vi "纳清叶绿素a电极校准.vi"() -> ()   [LabVIEW 2016, in "斯坦道多参数.lvlib"]
uses:
  <vilib>/Utility/miscctls.llb/LVPointTypeDef.ctl
  <vilib>/Utility/miscctls.llb/LVPositionTypeDef.ctl
  <vilib>/Analysis/NI_AALBase.lvlib
panel:
  out "温度校准参数":sgl
  out "第三点校准值":dbl
  out "标液3":sgl
  out "第二点校准值":dbl
  out "第一点校准值":dbl
  in  "校准停止":bool
  in  "校准启动":bool
  in  "校准模式":enum16{"两点校准", "单点校准", "三点校准"}(ring)=enum."单点校准"
  out "最小值":sgl format="%#.2f"
  out "最大值":sgl format="%#.2f"
  out "波形图表":u16(graph) caption="历史曲线"
  out "mean":dbl caption="均值" format="%#.2f"
  out "standard deviation":dbl caption="标准差" format="%#.2f"
  out "变异系数":dbl format="%#.6f"
  out "测量值":sgl
  out "提示":string
  out "标液2":sgl
  out "标液1":sgl
  out "原始光强数值":u16 caption="信号值"
  out "温度":dbl
  # "叶绿素a电极设定"
  # "℃"
  # "ug/L"
  # "℃"
  # "请选择校准模式:"
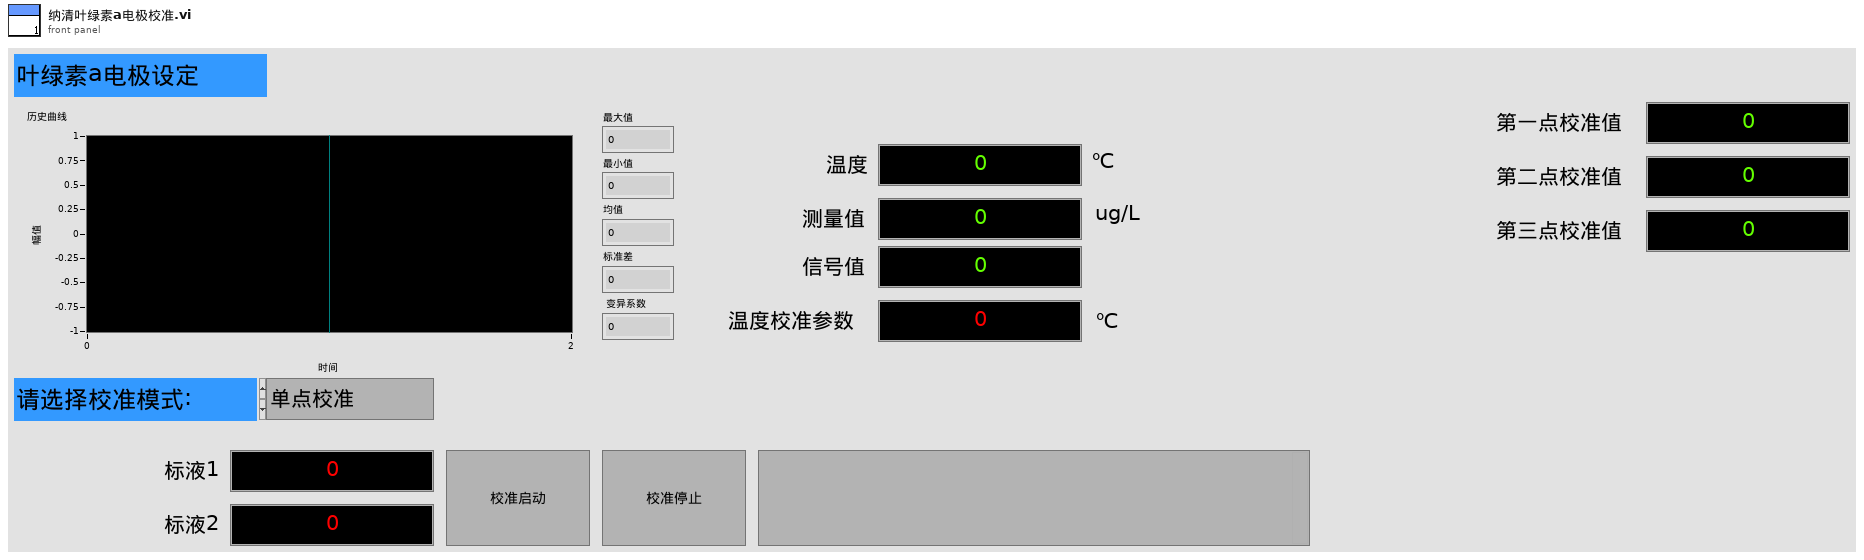
[diagram p1: front panel]
types:
  T1 = typedef "LVPointTypeDef.ctl" = cluster{"Horizontal":i16, "Vertical":i16}
  T2 = typedef "斯坦道多参数.lvlib/校准步骤.ctl" = enum16{"待机", "放置第一点标液", "第一点校准启动", "第一点校准写入", "第一点校准失败", "放置第二点标液", "第二点校准启动", "第二点校准写入", "第二点校准失败", "放置第三点标液", "第三点校准启动", "第三点校准写入", "第三点校准失败", "校准结果写入", "校准结束"}
  T3 = cluster{"报警码":u16, "叶绿素a":sgl, "温度数据":sgl, "原始光强数值":u16, "0X0006_NC":u16, "平均次数":u16, "清扫模式":u16, "清扫次数":u16, "清扫间隔分钟":u16, "0X000B_NC":string, "产品名称":string, "序列号":string, "硬件版本":string, "软件版本":string, "通讯地址":u16, "波特率":u16, "设备类型":u16, "0X0026_NC":string, "0X0030_NC":u16, "第一点原始光强":u16, "第一点校准数据":sgl, "第二点原始光强":u16, "第二点校准数据":sgl, "第三点原始光强":u16, "第三点校准数据":sgl, "探头校准命令":u16, "温度校准参数":sgl, "温度校准命令":u16}
  T4 = typedef "LVPositionTypeDef.ctl" = cluster{"Left":i32, "Top":i32}
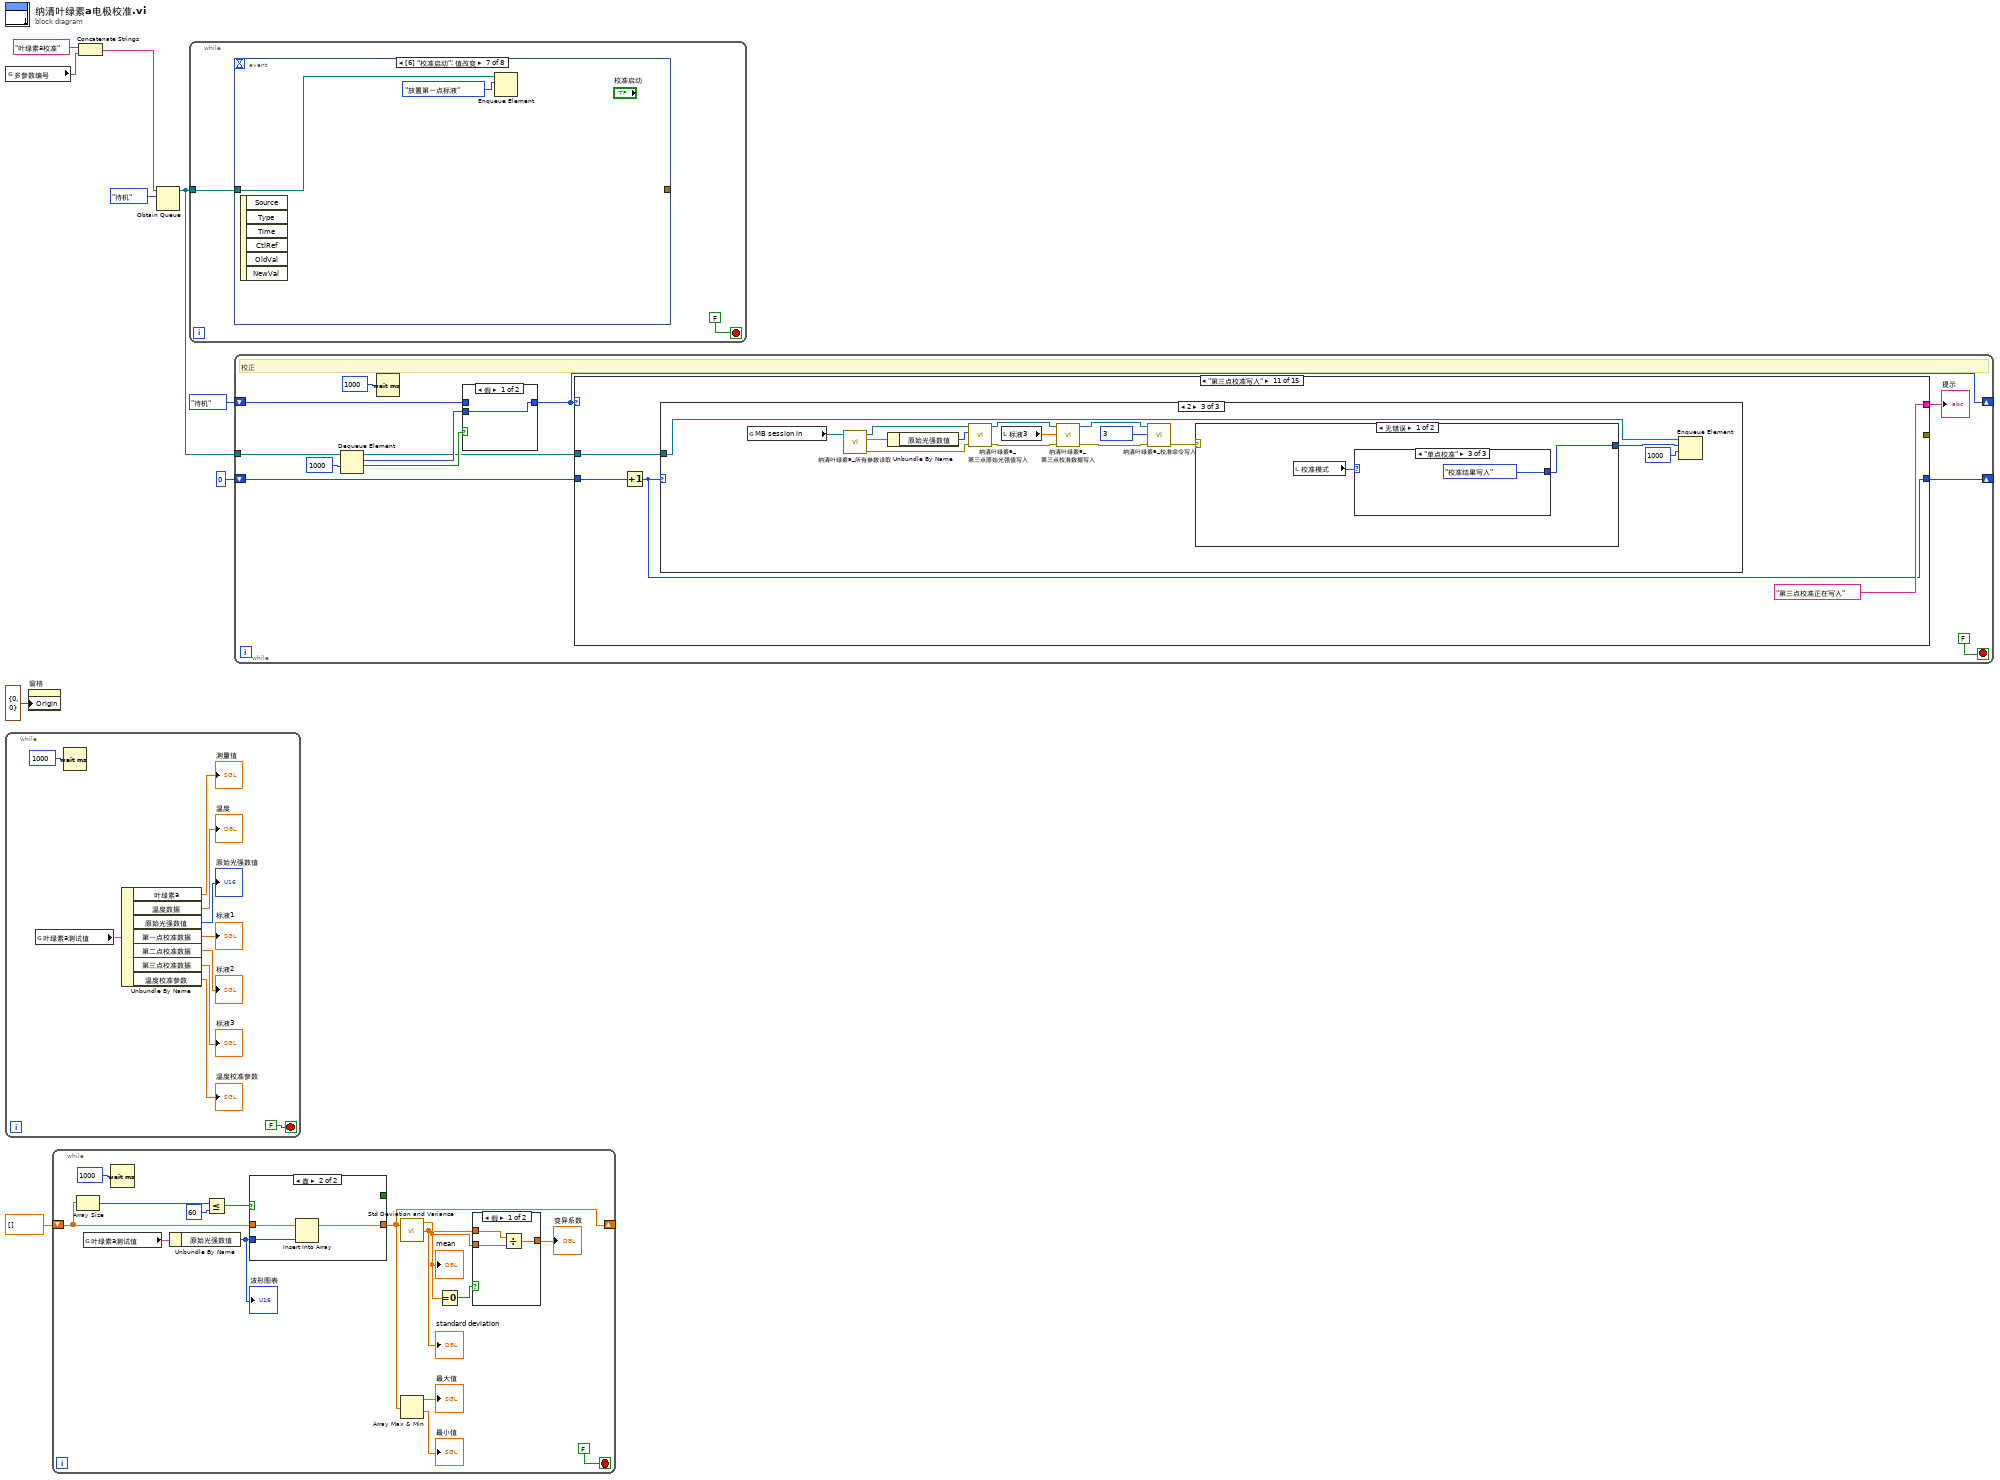
[diagram p0: block diagram]
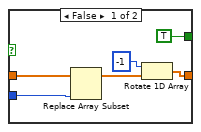
[diagram p3: hidden frame]
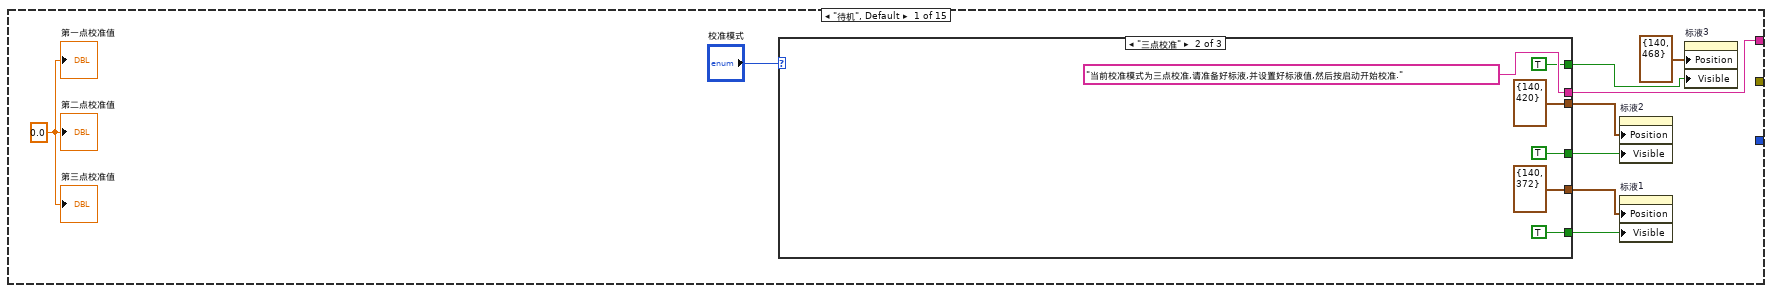
[diagram p5: hidden frame]
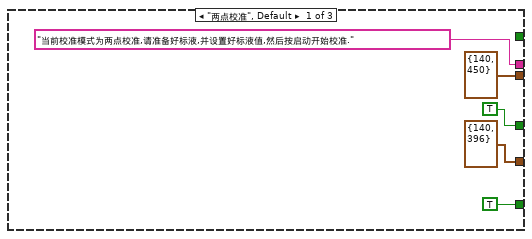
[diagram p6: hidden frame]
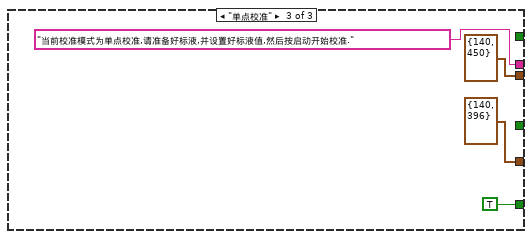
[diagram p7: hidden frame]
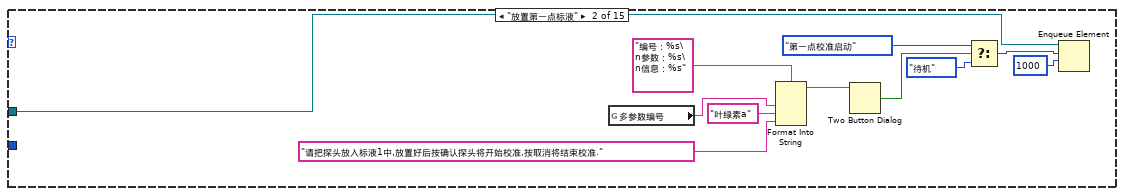
[diagram p8: hidden frame]
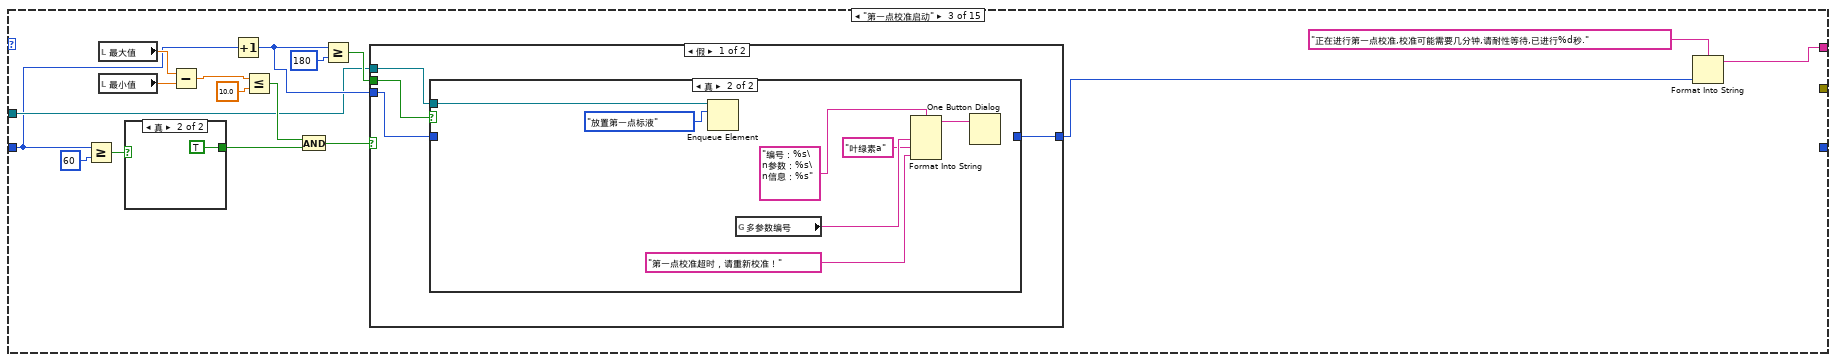
[diagram p9: hidden frame]
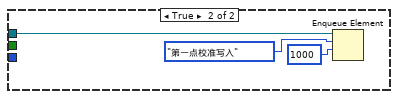
[diagram p11: hidden frame]
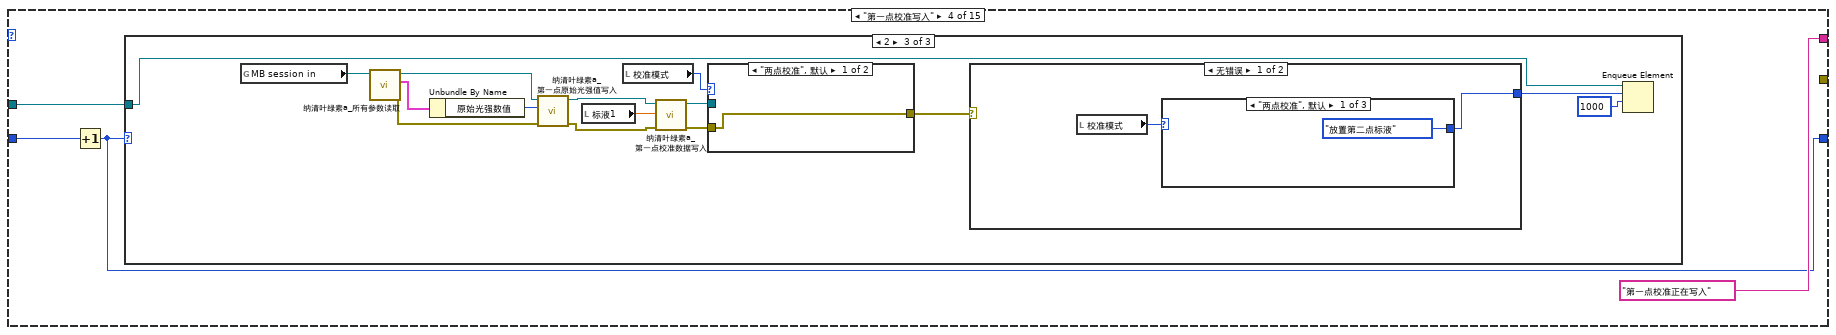
[diagram p13: hidden frame]
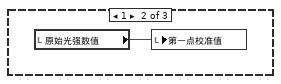
[diagram p15: hidden frame]
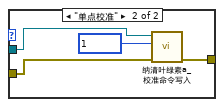
[diagram p16: hidden frame]
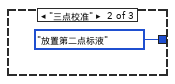
[diagram p17: hidden frame]
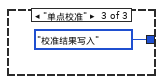
[diagram p18: hidden frame]
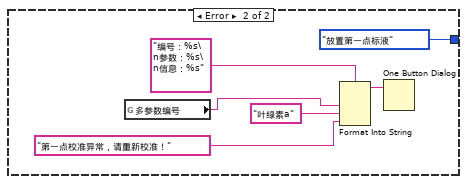
[diagram p19: hidden frame]
diagram:
  n1 = global read "多参数全局变量.vi" "多参数编号"() -> (w1:string)
  n2 = while {
    stop <- FALSE stop-if-true
    n3 = global read "纳清过程全局变量.vi" "叶绿素a测试值"() -> (w17:T3)
    n4 = Wait (ms)(milliseconds to wait=u32 1000 ("等待时间（毫秒）")) -> ()  [unwired: 1 out]
    n5 = Unbundle By Name(w17) -> ("叶绿素a"=→"测量值":sgl, "温度数据"=→"温度":sgl, "原始光强数值"=→"原始光强数值":u16, "第一点校准数据"=→"标液1":sgl, "第二点校准数据"=→"标液2":sgl, "第三点校准数据"=→"标液3":sgl, "温度校准参数"=→"温度校准参数":sgl)
  }
  n6 = property on="窗格" class="Pane"("Origin"=T1 {"Horizontal"=0, "Vertical"=0} ("原点")) -> ()  [unwired: 2 in, 2 out]
  n7 = while {
    shift-right: [w24] -> _
    shift-left: sgl[] [] -> [w30]
    stop <- FALSE stop-if-true
    n8 = Array Size(array=w30) -> (size(s)=w32:i32)
    n9 = global read "纳清过程全局变量.vi" "叶绿素a测试值"() -> (w20:T3)
    n10 = Wait (ms)(milliseconds to wait=u32 1000 ("等待时间（毫秒）")) -> ()  [unwired: 1 out]
    n11 = Unbundle By Name(w20) -> ("原始光强数值"=w21:u16)
    "波形图表" <- w21
    n12 = Less Or Equal?(x=w32, y=60) -> (x <= y?=w31:bool)
    n13 = case shown="真" w31 {
      tunnel: w30 -> [w43 w46]
      tunnel: w21 -> [w41 w45]
      tunnel: [w39 w44] -> w24
      tunnel: [TRUE _] -> _
      frame False {
        n14 = Replace Array Subset(array=w43, new element=w41) -> (w42:sgl[])  [unwired: 1 in]
        n15 = Rotate 1D Array(1:w42, 2:-1 ("n")) -> (0:w39:sgl[])
      }
      frame True {
        n16 = Insert Into Array(array=w46, new element=w45) -> (w44:sgl[])  [unwired: 1 in]
      }
    }
    n17 = call <vilib>:"Std Deviation and Variance.vi"("X"=w24) -> ("mean"=w28:dbl, "standard deviation"=w27:dbl)  [unwired: 1 in, 1 out]
    "mean" <- w28
    "standard deviation" <- w27
    n18 = Array Max & Min(array=w24) -> (max value=→"最大值":sgl, min value=→"最小值":sgl)  [unwired: 2 out]
    n19 = Equal To 0?(x=w28) -> (x = 0?=w29:bool)
    n20 = case shown="假" w29 {
      tunnel: w27 -> [w37 _]
      tunnel: [w36 _] -> w26
      tunnel: w28 -> [w35 _]
      frame False {
        n21 = Divide(x=w37, y=w35) -> (x/y=w36:dbl)
      }
      frame True {
      }
    }
    "变异系数" <- w26
  }
  n22 = Concatenate Strings("叶绿素a校准" ("名称（未命名）"), w1) -> (w2:string)
  n23 = Obtain Queue(name (unnamed)=w2, element data type=校准步骤."待机" ("枚举")) -> (queue out=w4:refnum<queue>)  [unwired: 3 in, 2 out]
  n24 = while {
    tunnel: w4 -> [w47]
    stop <- FALSE stop-if-true
    n25 = event shown="[6] \"校准启动\": 值改变" {
      selector: _ -> [_ _ _ _ _ _ _ _]
      dyn-events: _ -> [_ _ _ _ _ _ _ _]
      timeout: _ -> [_ _ _ _ _ _ _ _]
      tunnel: [_ _ w54 w58 w61 w62 _ _] -> _
      tunnel: w47 -> [_ _ _ _ _ _ w69 w71]
      event Timeout {
        n26 = event-data() -> ()  [unwired: 1 in, 3 out]
      }
      event "标液1", "标液2", "标液3", "温度校准参数": Mouse Down {
        n27 = event-data() -> ("CtlRef"=w49:refnum<vi>)  [unwired: 1 in, 7 out]
        n28 = property class="DigNum (严格)"(reference=w49) -> (reference out=w50:refnum<vi>, "Value"=w51:sgl)  [unwired: 1 in, 1 out]
        n29 = call "数字键盘.vi"("OldNumber"=w51) -> ("NewNumber"=w52:dbl)  [unwired: 1 in]
        n30 = property class="DigNum (严格)"(reference=w50, "Val(Sgnl)"=w52) -> ()  [unwired: 1 in, 2 out]
      }
      event "标液1": Value Change {
        n31 = event-data() -> ("NewVal"=w53:sgl)  [unwired: 1 in, 5 out]
        n32 = global read "多参数全局变量.vi" "MB session in"() -> (w55:refnum<class "MB_Master.lvclass">)
        n33 = call "纳清叶绿素a_第一点校准数据写入.vi"("数值"=w53, "MB session in"=w55) -> ("error out"=w54:errorcluster)  [unwired: 8 in, 1 out]
      }
      event "标液2": Value Change {
        n34 = event-data() -> ("NewVal"=w57:sgl)  [unwired: 1 in, 5 out]
        n35 = global read "多参数全局变量.vi" "MB session in"() -> (w56:refnum<class "MB_Master.lvclass">)
        n36 = call "纳清叶绿素a_第二点校准数据写入.vi"("数值"=w57, "MB session in"=w56) -> ("error out"=w58:errorcluster)  [unwired: 8 in, 1 out]
      }
      event "标液3": Value Change {
        n37 = event-data() -> ("NewVal"=w59:sgl)  [unwired: 1 in, 5 out]
        n38 = global read "多参数全局变量.vi" "MB session in"() -> (w60:refnum<class "MB_Master.lvclass">)
        n39 = call "纳清叶绿素a_第三点校准数据写入.vi"("数值"=w59, "MB session in"=w60) -> ("error out"=w61:errorcluster)  [unwired: 8 in, 1 out]
      }
      event "温度校准参数": Value Change {
        n40 = event-data() -> ("NewVal"=w67:sgl)  [unwired: 1 in, 5 out]
        n41 = global read "多参数全局变量.vi" "MB session in"() -> (w66:refnum<class "MB_Master.lvclass">)
        n42 = call "纳清叶绿素a_温度校准参数写入.vi"("数值"=w67, "MB session in"=w66) -> ("error out"=w68:errorcluster, "MB session out"=w65:refnum<class "MB_Master.lvclass">)  [unwired: 8 in]
        n43 = call "纳清叶绿素a_温度校准命令写入.vi"("error in (no error)"=w68, "数值"=u16 1 ("starting address"), "MB session in"=w65) -> ("error out"=w63:errorcluster)  [unwired: 7 in, 1 out]
        n44 = call <vilib>:"Simple Error Handler.vi"("error in (no error)"=w63) -> ("error out"=w62:errorcluster)  [unwired: 4 in, 4 out]
      }
      event "校准启动": Value Change {
        n45 = event-data() -> ()  [unwired: 1 in, 6 out]
        n46 = Enqueue Element(queue=w69, element=校准步骤."放置第一点标液" ("元素")) -> ()  [unwired: 2 in, 3 out]
      }
      event "校准停止": Value Change {
        n47 = event-data() -> ()  [unwired: 1 in, 6 out]
        n48 = Flush Queue(queue=w71) -> (queue out=w72:refnum<queue>)  [unwired: 1 in, 2 out]
        n49 = Enqueue Element(queue=w72, element=校准步骤."待机" ("元素"), timeout in ms (-1)=1000 ("超时毫秒(-1)")) -> ()  [unwired: 1 in, 3 out]
      }
    }
  }
  n50 = while "While循环" {
    shift-right: [w76] -> _
    shift-left: 校准步骤."待机" ("枚举") -> [w78]
    shift-right: [w75] -> _
    shift-left: 0 -> [w84]
    tunnel: w4 -> [w79]
    stop <- FALSE stop-if-true
    # "校正"
    n51 = Dequeue Element(queue=w79, timeout in ms (-1)=1000 ("超时毫秒(-1)")) -> (queue out=w77:refnum<queue>, element=w80:T2, timed out?=w81:bool)  [unwired: 1 in, 1 out]
    n52 = Wait (ms)(milliseconds to wait=u32 1000 ("等待时间（毫秒）")) -> ()  [unwired: 1 out]
    n53 = case shown="假" w81 {
      tunnel: w80 -> [w87 _]
      tunnel: [w87 w88] -> w76
      tunnel: w78 -> [_ w88]
      frame False {
      }
      frame True {
      }
    }
    n54 = case shown="\"第三点校准写入\"" w76 {
      tunnel: [w96 _ w124 "第一点校准正在写入" ("提示") _ _ w206 "第二点校准正在写入" ("提示") "第二点校准失败" ("提示") _ "第三点校准正在写入" ("提示") w318 "第三点校准失败" ("提示") w350 w377] -> w83
      tunnel: w84 -> [_ _ w126 w159 _ _ w207 w239 _ _ w287 w319 _ _ _]
      tunnel: [_ _ _ w157 _ _ w205 w237 _ _ w285 w317 _ _ _] -> w75
      tunnel: w77 -> [_ w119 w127 w158 _ w198 w208 w238 _ w279 w286 w320 _ w357 _]
      tunnel: [_ _ _ _ _ _ _ _ _ _ _ _ _ w355 _] -> _
      frame "待机", Default {
        w89 = 0.0 ("第一点校准值")
        n55 = case shown="\"三点校准\"" "校准模式" {
          tunnel: ["当前校准模式为两点校准,请准备好标液,并设置好标液值,然后按启动开始校准." ("提示") "当前校准模式为三点校准,请准备好标液,并设置好标液值,然后按启动开始校准." ("提示") "当前校准模式为单点校准,请准备好标液,并设置好标液值,然后按启动开始校准." ("提示")] -> w96
          tunnel: [TRUE ("可见") TRUE ("可见") _] -> w92
          tunnel: [T4 {"Left"=140, "Top"=396} ("位置") T4 {"Left"=140, "Top"=372} ("位置") T4 {"Left"=140, "Top"=396} ("位置")] -> w95
          tunnel: [T4 {"Left"=140, "Top"=450} ("位置 2") T4 {"Left"=140, "Top"=420} ("位置 2") T4 {"Left"=140, "Top"=450} ("位置 2")] -> w94
          tunnel: [_ TRUE ("可见") _] -> w91
          tunnel: [TRUE ("可见") TRUE ("可见") TRUE ("可见")] -> w90
          frame "两点校准", Default {
          }
          frame "三点校准" {
          }
          frame "单点校准" {
          }
        }
        n56 = property on="标液2" class="DigNum (严格)"("Position"=w94, "Visible"=w92) -> ()  [unwired: 2 in, 2 out]
        n57 = property on="标液1" class="DigNum (严格)"("Position"=w95, "Visible"=w90) -> ()  [unwired: 2 in, 2 out]
        n58 = property on="标液3" class="DigNum (严格)"("Position"=T4 {"Left"=140, "Top"=468} ("位置 3"), "Visible"=w91) -> ()  [unwired: 2 in, 2 out]
        "第一点校准值" <- w89
        "第二点校准值" <- w89
        "第三点校准值" <- w89
      }
      frame "放置第一点标液" {
        n59 = global read "多参数全局变量.vi" "多参数编号"() -> (w117:string)
        n60 = Format Into String(format string="编号：%s\n参数：%s\n信息：%s" ("格式字符串"), w117, "叶绿素a" ("输入 2"), "请把探头放入标液1中,放置好后按确认探头将开始校准,按取消将结束校准." ("消息")) -> (resulting string=w115:string)  [unwired: 2 in, 1 out]
        n61 = Two Button Dialog(message=w115) -> (T button?=w113:bool)  [unwired: 2 in]
        n62 = Select(t=校准步骤."第一点校准启动" ("元素"), s=w113, f=校准步骤."待机" ("元素")) -> (s? t:f=w120:T2)
        n63 = Enqueue Element(queue=w119, element=w120, timeout in ms (-1)=1000 ("超时毫秒(-1)")) -> ()  [unwired: 1 in, 3 out]
      }
      frame "第一点校准启动" {
        n64 = Greater Or Equal?(x=w126, y=60) -> (x >= y?=w133:bool)
        n65 = local read "最大值"() -> (w136:sgl)
        n66 = local read "最小值"() -> (w135:sgl)
        n67 = case shown="真" w133 {
          tunnel: [_ TRUE] -> w134
          frame False {
          }
          frame True {
          }
        }
        n68 = Subtract(x=w136, y=w135) -> (x-y=w137:sgl)
        n69 = Increment(x=w126) -> (x+1=w140:i32)
        n70 = Less Or Equal?(x=w137, y=10.0) -> (x <= y?=w130:bool)
        n71 = And(x=w130, y=w134) -> (x .and. y?=w138:bool)
        n72 = Greater Or Equal?(x=w140, y=180) -> (x >= y?=w139:bool)
        n73 = case shown="假" w138 {
          tunnel: w127 -> [w143 w155]
          tunnel: w139 -> [w144 _]
          tunnel: w140 -> [w142 _]
          tunnel: [w141 _] -> w125
          frame False {
            n74 = case shown="真" w144 {
              tunnel: w143 -> [_ w152]
              tunnel: w142 -> [w145 _]
              tunnel: [w145 _] -> w141
              frame False {
              }
              frame True {
                n75 = Enqueue Element(queue=w152, element=校准步骤."放置第一点标液" ("元素")) -> ()  [unwired: 2 in, 3 out]
                n76 = global read "多参数全局变量.vi" "多参数编号"() -> (w149:string)
                n77 = Format Into String(format string="编号：%s\n参数：%s\n信息：%s" ("格式字符串"), w149, "叶绿素a" ("输入 2"), "第一点校准超时，请重新校准！" ("error source (\" \")")) -> (resulting string=w146:string)  [unwired: 2 in, 1 out]
                n78 = One Button Dialog(message=w146) -> ()  [unwired: 1 in, 1 out]
              }
            }
          }
          frame True {
            n79 = Enqueue Element(queue=w155, element=校准步骤."第一点校准写入" ("元素"), timeout in ms (-1)=1000 ("超时毫秒(-1)")) -> ()  [unwired: 1 in, 3 out]
          }
        }
        n80 = Format Into String(format string="正在进行第一点校准,校准可能需要几分钟,请耐性等待,已进行%d秒." ("格式字符串"), w125) -> (resulting string=w124:string)  [unwired: 2 in, 1 out]
      }
      frame "第一点校准写入" {
        n81 = Increment(x=w159) -> (x+1=w157:i32)
        n82 = case shown="2" w157 {
          tunnel: w158 -> [_ _ w176]
          frame 0, Default {
          }
          frame 1 {
            n83 = local read "原始光强数值"() -> (w161:u16)
            n84 = local write "第一点校准值"(w161) -> ()
          }
          frame 2 {
            n85 = global read "多参数全局变量.vi" "MB session in"() -> (w172:refnum<class "MB_Master.lvclass">)
            n86 = call "纳清叶绿素a_所有参数读取.vi"("MB session in"=w172) -> ("error out"=w174:errorcluster, "输出值"=w171:T3, "MB session out"=w173:refnum<class "MB_Master.lvclass">)  [unwired: 8 in]
            n87 = Unbundle By Name(w171) -> ("原始光强数值"=w170:u16)
            n88 = call "纳清叶绿素a_第一点原始光强值写入.vi"("error in (no error)"=w174, "数值"=w170, "MB session in"=w173) -> ("error out"=w169:errorcluster, "MB session out"=w168:refnum<class "MB_Master.lvclass">)  [unwired: 7 in]
            n89 = local read "标液1"() -> (w165:sgl)
            n90 = local read "校准模式"() -> (w162:enum16{"两点校准", "单点校准", "三点校准"})
            n91 = call "纳清叶绿素a_第一点校准数据写入.vi"("error in (no error)"=w169, "数值"=w165, "MB session in"=w168) -> ("error out"=w167:errorcluster, "MB session out"=w166:refnum<class "MB_Master.lvclass">)  [unwired: 7 in]
            n92 = case shown="\"两点校准\", 默认" w162 {
              tunnel: w167 -> [w177 w181]
              tunnel: w166 -> [_ w180]
              tunnel: [w177 w178] -> w164
              frame "两点校准", Default {
              }
              frame "单点校准" {
                n93 = call "纳清叶绿素a_校准命令写入.vi"("error in (no error)"=w181, "数值"=u16 1 ("starting address"), "MB session in"=w180) -> ("error out"=w178:errorcluster)  [unwired: 7 in, 1 out]
              }
            }
            n94 = case shown="无错误" w164 {
              tunnel: [w182 校准步骤."放置第一点标液" ("元素")] -> w163
              frame No Error {
                n95 = local read "校准模式"() -> (w183:enum16{"两点校准", "单点校准", "三点校准"})
                n96 = case shown="\"两点校准\", 默认" w183 {
                  tunnel: [校准步骤."放置第二点标液" ("元素") 校准步骤."放置第二点标液" ("元素") 校准步骤."校准结果写入" ("元素")] -> w182
                  frame "两点校准", Default {
                  }
                  frame "三点校准" {
                  }
                  frame "单点校准" {
                  }
                }
              }
              frame Error {
                n97 = global read "多参数全局变量.vi" "多参数编号"() -> (w191:string)
                n98 = Format Into String(format string="编号：%s\n参数：%s\n信息：%s" ("格式字符串"), w191, "叶绿素a" ("输入 2"), "第一点校准异常，请重新校准！" ("error source (\" \")")) -> (resulting string=w188:string)  [unwired: 2 in, 1 out]
                n99 = One Button Dialog(message=w188) -> ()  [unwired: 1 in, 1 out]
              }
            }
            n100 = Enqueue Element(queue=w176, element=w163, timeout in ms (-1)=1000 ("超时毫秒(-1)")) -> ()  [unwired: 1 in, 3 out]
          }
        }
      }
      frame "第一点校准失败" {
      }
      frame "放置第二点标液" {
        n101 = global read "多参数全局变量.vi" "多参数编号"() -> (w196:string)
        n102 = Format Into String(format string="编号：%s\n参数：%s\n信息：%s" ("格式字符串"), w196, "叶绿素a" ("输入 2"), "请把探头放入标液2中,放置好后按确认将继续校准,按取消将结束校准." ("消息")) -> (resulting string=w194:string)  [unwired: 2 in, 1 out]
        n103 = Two Button Dialog(message=w194) -> (T button?=w202:bool)  [unwired: 2 in]
        n104 = Select(t=校准步骤."第二点校准启动" ("元素"), s=w202, f=校准步骤."待机" ("元素")) -> (s? t:f=w199:T2)
        n105 = Enqueue Element(queue=w198, element=w199, timeout in ms (-1)=1000 ("超时毫秒(-1)")) -> ()  [unwired: 1 in, 3 out]
      }
      frame "第二点校准启动" {
        n106 = Greater Or Equal?(x=w207, y=60) -> (x >= y?=w213:bool)
        n107 = local read "最大值"() -> (w216:sgl)
        n108 = local read "最小值"() -> (w215:sgl)
        n109 = case shown="真" w213 {
          tunnel: [_ TRUE] -> w214
          frame False {
          }
          frame True {
          }
        }
        n110 = Subtract(x=w216, y=w215) -> (x-y=w217:sgl)
        n111 = Increment(x=w207) -> (x+1=w220:i32)
        n112 = Less Or Equal?(x=w217, y=10.0) -> (x <= y?=w210:bool)
        n113 = And(x=w210, y=w214) -> (x .and. y?=w218:bool)
        n114 = Greater Or Equal?(x=w220, y=180) -> (x >= y?=w219:bool)
        n115 = case shown="假" w218 {
          tunnel: w208 -> [w223 w235]
          tunnel: w219 -> [w224 _]
          tunnel: w220 -> [w222 _]
          tunnel: [w221 _] -> w205
          frame False {
            n116 = case shown="真" w224 {
              tunnel: w223 -> [_ w232]
              tunnel: w222 -> [w225 _]
              tunnel: [w225 _] -> w221
              frame False {
              }
              frame True {
                n117 = Enqueue Element(queue=w232, element=校准步骤."放置第二点标液" ("元素")) -> ()  [unwired: 2 in, 3 out]
                n118 = global read "多参数全局变量.vi" "多参数编号"() -> (w229:string)
                n119 = Format Into String(format string="编号：%s\n参数：%s\n信息：%s" ("格式字符串"), w229, "叶绿素a" ("输入 2"), "第二点校准超时，请重新校准！" ("消息")) -> (resulting string=w227:string)  [unwired: 2 in, 1 out]
                n120 = One Button Dialog(message=w227) -> ()  [unwired: 1 in, 1 out]
              }
            }
          }
          frame True {
            n121 = Enqueue Element(queue=w235, element=校准步骤."第二点校准写入" ("元素"), timeout in ms (-1)=1000 ("超时毫秒(-1)")) -> ()  [unwired: 1 in, 3 out]
          }
        }
        n122 = Format Into String(format string="正在进行第二点校准,校准可能需要几分钟,请耐性等待,已进行%d秒." ("格式字符串"), w205) -> (resulting string=w206:string)  [unwired: 2 in, 1 out]
      }
      frame "第二点校准写入" {
        n123 = Increment(x=w239) -> (x+1=w237:i32)
        n124 = case shown="2" w237 {
          tunnel: w238 -> [_ _ w256]
          frame 0, Default {
          }
          frame 1 {
            n125 = local read "原始光强数值"() -> (w241:u16)
            n126 = local write "第二点校准值"(w241) -> ()
          }
          frame 2 {
            n127 = global read "多参数全局变量.vi" "MB session in"() -> (w252:refnum<class "MB_Master.lvclass">)
            n128 = call "纳清叶绿素a_所有参数读取.vi"("MB session in"=w252) -> ("error out"=w254:errorcluster, "输出值"=w251:T3, "MB session out"=w253:refnum<class "MB_Master.lvclass">)  [unwired: 8 in]
            n129 = Unbundle By Name(w251) -> ("原始光强数值"=w250:u16)
            n130 = call "纳清叶绿素a_第二点原始光强值写入.vi"("error in (no error)"=w254, "数值"=w250, "MB session in"=w253) -> ("error out"=w249:errorcluster, "MB session out"=w248:refnum<class "MB_Master.lvclass">)  [unwired: 7 in]
            n131 = local read "标液2"() -> (w245:sgl)
            n132 = local read "校准模式"() -> (w242:enum16{"两点校准", "单点校准", "三点校准"})
            n133 = call "纳清叶绿素a_第二点校准数据写入.vi"("error in (no error)"=w249, "数值"=w245, "MB session in"=w248) -> ("error out"=w247:errorcluster, "MB session out"=w246:refnum<class "MB_Master.lvclass">)  [unwired: 7 in]
            n134 = case shown="\"单点校准\", 默认" w242 {
              tunnel: w247 -> [w260 w261]
              tunnel: w246 -> [w259 _]
              tunnel: [w257 w261] -> w244
              frame "两点校准" {
                n135 = call "纳清叶绿素a_校准命令写入.vi"("error in (no error)"=w260, "数值"=u16 2 ("starting address"), "MB session in"=w259) -> ("error out"=w257:errorcluster)  [unwired: 7 in, 1 out]
              }
              frame "单点校准", Default {
              }
            }
            n136 = case shown="无错误" w244 {
              tunnel: [w262 校准步骤."放置第二点标液" ("元素")] -> w243
              frame No Error {
                n137 = local read "校准模式"() -> (w263:enum16{"两点校准", "单点校准", "三点校准"})
                n138 = case shown="\"两点校准\", 默认" w263 {
                  tunnel: [校准步骤."校准结果写入" ("元素") 校准步骤."放置第三点标液" ("元素") 校准步骤."校准结果写入" ("元素")] -> w262
                  frame "两点校准", Default {
                  }
                  frame "三点校准" {
                  }
                  frame "单点校准" {
                  }
                }
              }
              frame Error {
                n139 = global read "多参数全局变量.vi" "多参数编号"() -> (w271:string)
                n140 = Format Into String(format string="编号：%s\n参数：%s\n信息：%s" ("格式字符串"), w271, "叶绿素a" ("输入 2"), "第二点校准异常，请重新校准！" ("error source (\" \")")) -> (resulting string=w268:string)  [unwired: 2 in, 1 out]
                n141 = One Button Dialog(message=w268) -> ()  [unwired: 1 in, 1 out]
              }
            }
            n142 = Enqueue Element(queue=w256, element=w243, timeout in ms (-1)=1000 ("超时毫秒(-1)")) -> ()  [unwired: 1 in, 3 out]
          }
        }
      }
      frame "第二点校准失败" {
      }
      frame "放置第三点标液" {
        n143 = global read "多参数全局变量.vi" "多参数编号"() -> (w277:string)
        n144 = Format Into String(format string="编号：%s\n参数：%s\n信息：%s" ("格式字符串"), w277, "叶绿素a" ("输入 2"), "请把探头放入标液3中,放置好后按确认将继续校准,按取消将结束校准." ("消息")) -> (resulting string=w275:string)  [unwired: 2 in, 1 out]
        n145 = Two Button Dialog(message=w275) -> (T button?=w283:bool)  [unwired: 2 in]
        n146 = Select(t=校准步骤."第三点校准启动" ("元素"), s=w283, f=校准步骤."待机" ("元素")) -> (s? t:f=w280:T2)
        n147 = Enqueue Element(queue=w279, element=w280, timeout in ms (-1)=1000 ("超时毫秒(-1)")) -> ()  [unwired: 1 in, 3 out]
      }
      frame "第三点校准写入" {
        n148 = Increment(x=w287) -> (x+1=w285:i32)
        n149 = case shown="2" w285 {
          tunnel: w286 -> [_ _ w291]
          frame 0, Default {
          }
          frame 1 {
            n150 = local read "原始光强数值"() -> (w289:u16)
            n151 = local write "第二点校准值"(w289) -> ()
          }
          frame 2 {
            n152 = global read "多参数全局变量.vi" "MB session in"() -> (w302:refnum<class "MB_Master.lvclass">)
            n153 = call "纳清叶绿素a_所有参数读取.vi"("MB session in"=w302) -> ("error out"=w304:errorcluster, "输出值"=w301:T3, "MB session out"=w303:refnum<class "MB_Master.lvclass">)  [unwired: 8 in]
            n154 = Unbundle By Name(w301) -> ("原始光强数值"=w300:u16)
            n155 = call "纳清叶绿素a_第三点原始光强值写入.vi"("error in (no error)"=w304, "数值"=w300, "MB session in"=w303) -> ("error out"=w299:errorcluster, "MB session out"=w298:refnum<class "MB_Master.lvclass">)  [unwired: 7 in]
            n156 = local read "标液3"() -> (w294:sgl)
            n157 = call "纳清叶绿素a_第三点校准数据写入.vi"("error in (no error)"=w299, "数值"=w294, "MB session in"=w298) -> ("error out"=w297:errorcluster, "MB session out"=w296:refnum<class "MB_Master.lvclass">)  [unwired: 7 in]
            n158 = call "纳清叶绿素a_校准命令写入.vi"("error in (no error)"=w297, "数值"=u16 3 ("starting address"), "MB session in"=w296) -> ("error out"=w293:errorcluster)  [unwired: 7 in, 1 out]
            n159 = case shown="无错误" w293 {
              tunnel: [w305 校准步骤."放置第三点标液" ("元素")] -> w290
              frame No Error {
                n160 = local read "校准模式"() -> (w306:enum16{"两点校准", "单点校准", "三点校准"})
                n161 = case shown="\"单点校准\"" w306 {
                  tunnel: [校准步骤."放置第二点标液" ("元素") 校准步骤."校准结果写入" ("元素") 校准步骤."校准结果写入" ("元素")] -> w305
                  frame "两点校准", Default {
                  }
                  frame "三点校准" {
                  }
                  frame "单点校准" {
                  }
                }
              }
              frame Error {
                n162 = global read "多参数全局变量.vi" "多参数编号"() -> (w314:string)
                n163 = Format Into String(format string="编号：%s\n参数：%s\n信息：%s" ("格式字符串"), w314, "叶绿素a" ("输入 2"), "第三点校准异常，请重新校准！" ("error source (\" \")")) -> (resulting string=w311:string)  [unwired: 2 in, 1 out]
                n164 = One Button Dialog(message=w311) -> ()  [unwired: 1 in, 1 out]
              }
            }
            n165 = Enqueue Element(queue=w291, element=w290, timeout in ms (-1)=1000 ("超时毫秒(-1)")) -> ()  [unwired: 1 in, 3 out]
          }
        }
      }
      frame "第三点校准启动" {
        n166 = Greater Or Equal?(x=w319, y=60) -> (x >= y?=w325:bool)
        n167 = local read "最大值"() -> (w328:sgl)
        n168 = local read "最小值"() -> (w327:sgl)
        n169 = case shown="真" w325 {
          tunnel: [_ TRUE] -> w326
          frame False {
          }
          frame True {
          }
        }
        n170 = Subtract(x=w328, y=w327) -> (x-y=w329:sgl)
        n171 = Increment(x=w319) -> (x+1=w332:i32)
        n172 = Less Or Equal?(x=w329, y=10.0) -> (x <= y?=w322:bool)
        n173 = And(x=w322, y=w326) -> (x .and. y?=w330:bool)
        n174 = Greater Or Equal?(x=w332, y=180) -> (x >= y?=w331:bool)
        n175 = case shown="假" w330 {
          tunnel: w320 -> [w335 w347]
          tunnel: w331 -> [w336 _]
          tunnel: w332 -> [w334 _]
          tunnel: [w333 _] -> w317
          frame False {
            n176 = case shown="真" w336 {
              tunnel: w335 -> [_ w344]
              tunnel: w334 -> [w337 _]
              tunnel: [w337 _] -> w333
              frame False {
              }
              frame True {
                n177 = Enqueue Element(queue=w344, element=校准步骤."放置第三点标液" ("元素")) -> ()  [unwired: 2 in, 3 out]
                n178 = global read "多参数全局变量.vi" "多参数编号"() -> (w341:string)
                n179 = Format Into String(format string="编号：%s\n参数：%s\n信息：%s" ("格式字符串"), w341, "叶绿素a" ("输入 2"), "第三点校准异常，请重新校准！" ("error source (\" \")")) -> (resulting string=w338:string)  [unwired: 2 in, 1 out]
                n180 = One Button Dialog(message=w338) -> ()  [unwired: 1 in, 1 out]
              }
            }
          }
          frame True {
            n181 = Enqueue Element(queue=w347, element=校准步骤."第三点校准写入" ("元素"), timeout in ms (-1)=1000 ("超时毫秒(-1)")) -> ()  [unwired: 1 in, 3 out]
          }
        }
        n182 = Format Into String(format string="正在进行第三点校准,校准可能需要几分钟,请耐性等待,已进行%d秒." ("格式字符串"), w317) -> (resulting string=w318:string)  [unwired: 2 in, 1 out]
      }
      frame "第三点校准失败" {
      }
      frame "校准结果写入" {
        n183 = local read "校准模式"() -> (w356:enum16{"两点校准", "单点校准", "三点校准"})
        n184 = case shown="\"单点校准\"" w356 {
          tunnel: [w361 w369 w376] -> w351
          frame "两点校准", Default {
            n185 = local read "第一点校准值"() -> (w364:dbl)
            n186 = local read "第二点校准值"() -> (w360:dbl)
            n187 = local read "标液1"() -> (w362:sgl)
            n188 = local read "标液2"() -> (w359:sgl)
            n189 = Format Into String(format string="校准结果：第一点校准值=%f，第一点标准值=%f,第二点校准值=%f，第二点标准值=%f." ("提示"), w364, w362, w360, w359) -> (resulting string=w361:string)  [unwired: 2 in, 1 out]
          }
          frame "三点校准" {
            n190 = local read "第一点校准值"() -> (w372:dbl)
            n191 = local read "第二点校准值"() -> (w368:dbl)
            n192 = local read "第三点校准值"() -> (w366:dbl)
            n193 = local read "标液1"() -> (w370:sgl)
            n194 = local read "标液2"() -> (w367:sgl)
            n195 = local read "标液3"() -> (w365:sgl)
            n196 = Format Into String(format string="校准结果：第一点校准值=%f，第一点标准值=%f,第二点校准值=%f，第二点标准值=%f,第三点校准值=%f，第三点标准值=%f." ("提示"), w372, w370, w368, w367, w366, w365) -> (resulting string=w369:string)  [unwired: 2 in, 1 out]
          }
          frame "单点校准" {
            n197 = local read "第一点校准值"() -> (w375:dbl)
            n198 = local read "标液1"() -> (w373:sgl)
            n199 = Format Into String(format string="校准结果：校准值=%f，标准值=%f。" ("提示"), w375, w373) -> (resulting string=w376:string)  [unwired: 2 in, 1 out]
          }
        }
        n200 = Enqueue Element(queue=w357, element=校准步骤."校准结束" ("元素")) -> ()  [unwired: 2 in, 3 out]
        n201 = global read "多参数全局变量.vi" "多参数编号"() -> (w353:string)
        n202 = Format Into String(format string="编号：%s\n参数：%s\n信息：%s" ("格式字符串"), w353, "叶绿素a" ("输入 2"), w351) -> (resulting string=w350:string)  [unwired: 2 in, 1 out]
        n203 = One Button Dialog(message=w350) -> ()  [unwired: 1 in, 1 out]
        n204 = call "操作日志.vi"("日志信息"=w350) -> ("error out"=w355:errorcluster)  [unwired: 10 in]
      }
      frame "校准结束" {
        n205 = local read "提示"() -> (w377:string)
      }
    }
    "提示" <- w83
  }
